vi "ExMove2Spectro.vi"() -> ()   [LabVIEW 2010]
panel:
  out "error out 2":errorcluster
  out "Current Wavelength 2":string
  in  "Increment Wavelength 2":dbl=50.0 format="%.2f"
  in  "End Wavelength 2":dbl=700.0 format="%.2f"
  in  "Start Wavelength 2":dbl format="%.2f"
  in  "Grating Speed 2":dbl=2000.0 min=1.0 step=1.0 format="%.2f"
  in  "Grating number 2":i16=1 min=1 max=100 step=1
  out "Current Wavelength":string
  in  "Increment Wavelength":dbl=50.0 format="%.2f"
  in  "End Wavelength":dbl=700.0 format="%.2f"
  in  "Start Wavelength":dbl format="%.2f"
  in  "Grating Speed":dbl=2000.0 min=1.0 step=1.0 format="%.2f"
  in  "Grating number":i16=1 min=1 max=100 step=1
  out "error out":errorcluster
  in  "error in (no error)":errorcluster
  # "NOTES:\nA properly configured spectometer .ini must be present in the LabVIEW folder for spectrograph operation.  This MUST be defined for 2 spectrographs.\n\nConsult the Toolkit documentation for more information on how to configure this file."
  # "ExMove2Spectro.vi\n(Normal Spectrograph via USB/COM port)\nThis VI is a simple example of how to setup and move 2 spectrographs in increments over a wavelength range."
  # "SPECTROGRAPH 2"
  # "SPECTROGRAPH 1"
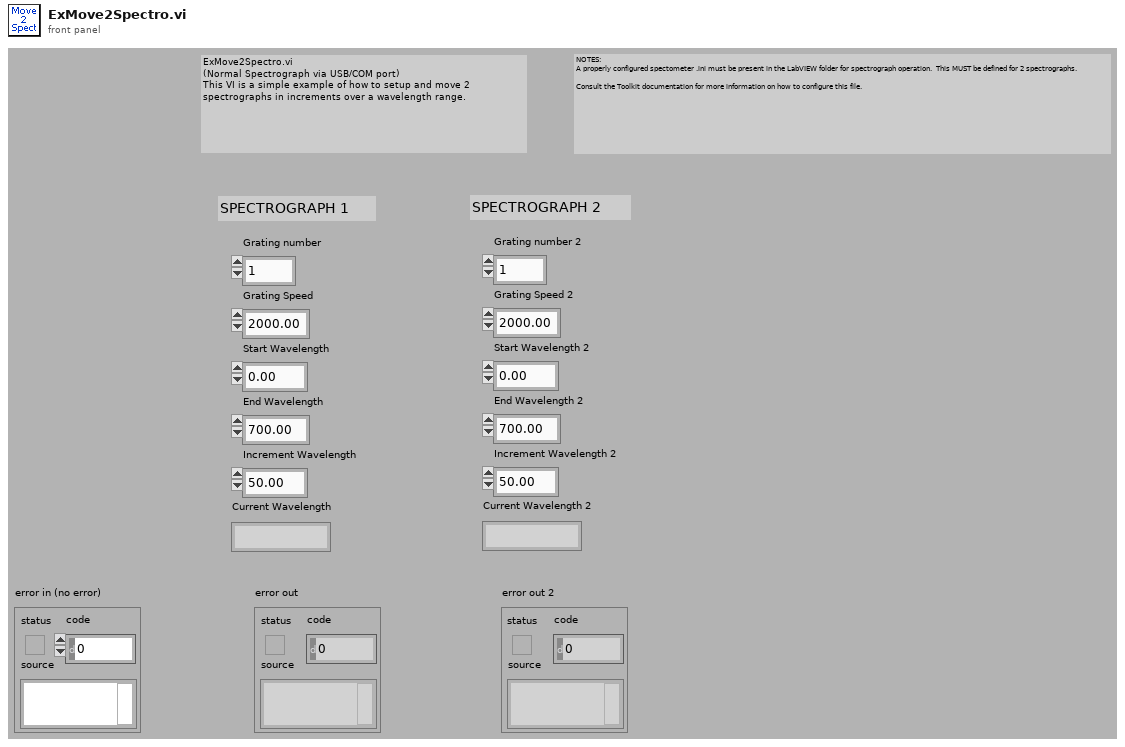
[diagram p1: front panel]
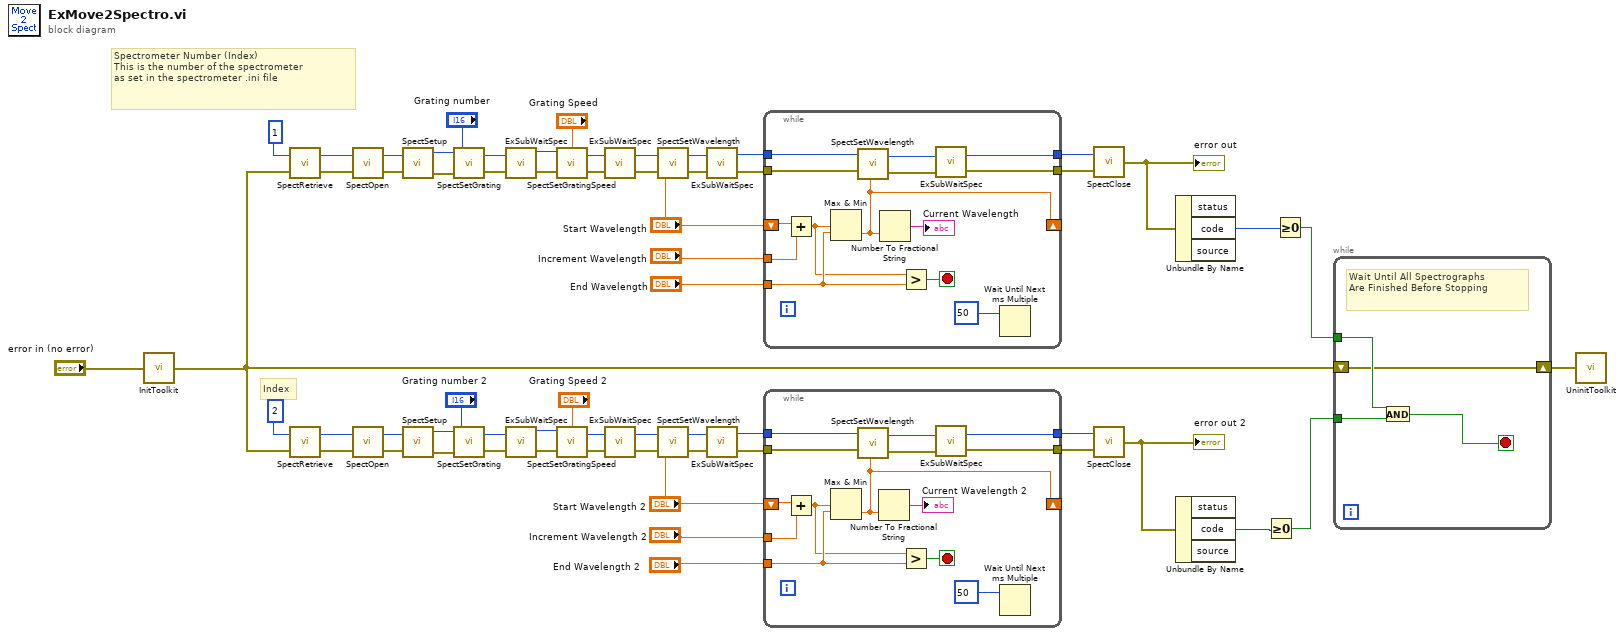
[diagram p0: block diagram]
diagram:
  # "Index"
  # "Spectrometer Number (Index)\nThis is the number of the spectrometer\nas set in the spectrometer .ini file"
  n1 = call <userlib>:"InitToolkit.vi"("error in"="error in (no error)") -> ("error out"=w6:errorcluster)
  n2 = call <userlib>:"SpectRetrieve.vi"("error in"=w6, "Index"=1) -> ("error out"=w39:errorcluster, "Device ID"=w38:u32)
  n3 = call <userlib>:"SpectRetrieve.vi"("error in"=w6, "Index"=2) -> ("error out"=w20:errorcluster, "Device ID"=w19:u32)
  n4 = call <userlib>:"SpectOpen.vi"("error in"=w39, "Spectrometer ID"=w38) -> ("error out"=w43:errorcluster, "Spectrometer Handle"=w45:u32)  [unwired: 1 in]
  n5 = call <userlib>:"SpectOpen.vi"("error in"=w20, "Spectrometer ID"=w19) -> ("error out"=w22:errorcluster, "Spectrometer Handle"=w24:u32)  [unwired: 1 in]
  n6 = call <userlib>:"SpectSetup.vi"("error in"=w43, "Spectrometer Handle"=w45) -> ("error out"=w42:errorcluster, "Spectrometer Handle"=w44:u32)
  n7 = call <userlib>:"SpectSetup.vi"("error in"=w22, "Spectrometer Handle"=w24) -> ("error out"=w21:errorcluster, "Spectrometer Handle"=w23:u32)
  n8 = call <userlib>:"SpectSetGrating.vi"("error in"=w42, "Grating Number"="Grating number", "Sepctrometer Handle"=w44) -> ("error out"=w51:errorcluster, "Spectrometer Handle"=w50:u32)
  n9 = call <userlib>:"SpectSetGrating.vi"("error in"=w21, "Grating Number"="Grating number 2", "Sepctrometer Handle"=w23) -> ("error out"=w30:errorcluster, "Spectrometer Handle"=w29:u32)
  n10 = call "ExSubWaitSpec.vi"("error in (no error)"=w51, "Spectrometer Handle"=w50) -> ("error out"=w49:errorcluster, "Spectrometer handle"=w48:u32)
  n11 = call "ExSubWaitSpec.vi"("error in (no error)"=w30, "Spectrometer Handle"=w29) -> ("error out"=w28:errorcluster, "Spectrometer handle"=w27:u32)
  n12 = call <userlib>:"SpectSetGratingSpeed.vi"("error in"=w49, "Grating Speed"="Grating Speed", "Spectrometer Handle"=w48) -> ("error out"=w46:errorcluster, "Spectrometer Handle"=w47:u32)
  n13 = call <userlib>:"SpectSetGratingSpeed.vi"("error in"=w28, "Grating Speed"="Grating Speed 2", "Spectrometer Handle"=w27) -> ("error out"=w25:errorcluster, "Spectrometer Handle"=w26:u32)
  n14 = call "ExSubWaitSpec.vi"("error in (no error)"=w46, "Spectrometer Handle"=w47) -> ("error out"=w36:errorcluster, "Spectrometer handle"=w37:u32)
  n15 = call "ExSubWaitSpec.vi"("error in (no error)"=w25, "Spectrometer Handle"=w26) -> ("error out"=w17:errorcluster, "Spectrometer handle"=w18:u32)
  n16 = call <userlib>:"SpectSetWavelength.vi"("error in"=w36, "Wavelength"="Start Wavelength", "Spectrometer Handle"=w37) -> ("error out"=w61:errorcluster, "Spectrumeter Handle"=w60:u32)
  n17 = call <userlib>:"SpectSetWavelength.vi"("error in"=w17, "Wavelength"="Start Wavelength 2", "Spectrometer Handle"=w18) -> ("error out"=w34:errorcluster, "Spectrumeter Handle"=w33:u32)
  n18 = call "ExSubWaitSpec.vi"("error in (no error)"=w61, "Spectrometer Handle"=w60) -> ("error out"=w53:errorcluster, "Spectrometer handle"=w59:u32)
  n19 = call "ExSubWaitSpec.vi"("error in (no error)"=w34, "Spectrometer Handle"=w33) -> ("error out"=w31:errorcluster, "Spectrometer handle"=w32:u32)
  n20 = while {
    tunnel: w59 -> [w66]
    tunnel: "Increment Wavelength" -> [w73]
    tunnel: "End Wavelength" -> [w65]
    shift-right: [w63] -> _
    shift-left: "Start Wavelength" -> [w74]
    tunnel: [w70] -> w55
    tunnel: [w67] -> w54
    tunnel: w53 -> [w69]
    stop <- w64 stop-if-true
    n21 = Add(x=w74, y=w73) -> (x+y=w62:dbl)
    n22 = Max & Min(x=w62, y=w65) -> (min(x,y)=w63:dbl)  [unwired: 1 out]
    n23 = call <userlib>:"SpectSetWavelength.vi"("error in"=w69, "Wavelength"=w63, "Spectrometer Handle"=w66) -> ("error out"=w68:errorcluster, "Spectrumeter Handle"=w71:u32)
    n24 = Number To Fractional String(number=w63) -> (F-format string=→"Current Wavelength":string)  [unwired: 3 in]
    n25 = Greater?(x=w62, y=w65) -> (0:w64:bool)
    n26 = call "ExSubWaitSpec.vi"("error in (no error)"=w68, "Spectrometer Handle"=w71) -> ("error out"=w67:errorcluster, "Spectrometer handle"=w70:u32)
    n27 = Wait Until Next ms Multiple(millisecond multiple=50) -> ()  [unwired: 1 out]
  }
  n28 = while {
    tunnel: w32 -> [w81]
    tunnel: "Increment Wavelength 2" -> [w87]
    tunnel: "End Wavelength 2" -> [w80]
    shift-right: [w78] -> _
    shift-left: "Start Wavelength 2" -> [w88]
    tunnel: [w85] -> w10
    tunnel: [w82] -> w9
    tunnel: w31 -> [w84]
    stop <- w79 stop-if-true
    n29 = Add(x=w88, y=w87) -> (x+y=w77:dbl)
    n30 = Max & Min(x=w77, y=w80) -> (min(x,y)=w78:dbl)  [unwired: 1 out]
    n31 = call <userlib>:"SpectSetWavelength.vi"("error in"=w84, "Wavelength"=w78, "Spectrometer Handle"=w81) -> ("error out"=w83:errorcluster, "Spectrumeter Handle"=w86:u32)
    n32 = Number To Fractional String(number=w78) -> (F-format string=→"Current Wavelength 2":string)  [unwired: 3 in]
    n33 = Greater?(x=w77, y=w80) -> (0:w79:bool)
    n34 = call "ExSubWaitSpec.vi"("error in (no error)"=w83, "Spectrometer Handle"=w86) -> ("error out"=w82:errorcluster, "Spectrometer handle"=w85:u32)
    n35 = Wait Until Next ms Multiple(millisecond multiple=50) -> ()  [unwired: 1 out]
  }
  n36 = call <userlib>:"SpectClose.vi"("error in"=w54, "Spectrometer Handle"=w55) -> ("error out"=w8:errorcluster)
  "error out" <- w8
  n37 = call <userlib>:"SpectClose.vi"("error in"=w9, "Spectrometer Handle"=w10) -> ("error out"=w3:errorcluster)
  "error out 2" <- w3
  n38 = Unbundle By Name(w8) -> ("code"=w7:i32)  [unwired: 2 out]
  n39 = Unbundle By Name(w3) -> ("code"=w2:i32)  [unwired: 2 out]
  n40 = Greater Or Equal To 0?(x=w2) -> (x >= 0?=w1:bool)
  n41 = Greater Or Equal To 0?(x=w7) -> (x >= 0?=w4:bool)
  n42 = while {
    shift-right: [w90] -> w5
    shift-left: w6 -> [w90]
    tunnel: w4 -> [w93]
    tunnel: w1 -> [w92]
    stop <- w91 stop-if-true
    # "Wait Until All Spectrographs\nAre Finished Before Stopping"
    n43 = And(x=w93, y=w92) -> (x .and. y?=w91:bool)
  }
  n44 = call <userlib>:"UninitToolkit.vi"("error in"=w5) -> ()  [unwired: 1 out]
